vi "IS PolyVI Instance Bool To JSON Cluster .vi"(3 "Stream Time (optional)":timestamp=timestamp(1451714400 s since 1904-01-01), 4 "Stream Value":bool, 5 "Stream Key":string) -> (1 "JSON Cluster Array out":T1[](array[typedef]))   [LabVIEW 2017]
uses:
  Custom Data Types/IS Data Point TypeDef (String).ctl
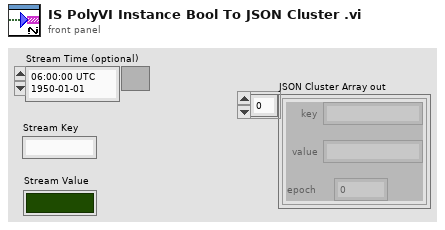
[diagram p1: front panel]
types:
  T1 = typedef "IS Data Point TypeDef (String).ctl" = cluster{"key":string, "value":string, "epoch":dbl}
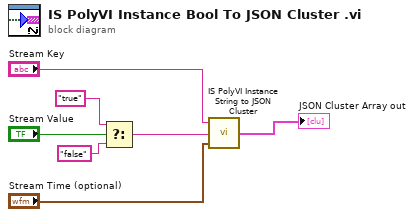
[diagram p0: block diagram]
diagram:
  n1 = Select(t="true", s="Stream Value", f="false") -> (s? t:f=w1:string)
  n2 = call "IS PolyVI Instance String to JSON Cluster.vi"("Stream Time (optional)"="Stream Time (optional)", "Stream Value"=w1, "Stream Key"="Stream Key") -> ("JSON Cluster Array out"=→"JSON Cluster Array out":T1[])  [unwired: 2 in]
